vi "GlobalArm.vi"() -> ()   [LabVIEW 2020]
uses:
  <vilib>/robotics/Kinematics/Robot/NI_Robotics_Serial Robot Arm.lvclass
panel:
  out "SEN_Current_Wrist_Angle (deg)":dbl
  out "SEN_Current_Shoulder_Angle (deg)":dbl
  out "SEN_Current_Elbow_Angle (deg)":dbl
  out "OUT_Arm_Goal_Position (in)":dbl[](array[numeric])=[1.35, 0.0, 0.0]
  out "CON_Arm_Base_Position (in)":dbl[](array[numeric])=[1.35, 0.0, 0.0]
  out "CON_Gripper_Cone_Center_Of_Gravity (in)":dbl[](array[numeric])=[1.35, 0.0, 0.0]
  out "CON_Gripper_None_Center_Of_Gravity (in)":dbl[](array[numeric])=[1.35, 0.0, 0.0]
  out "CON_Forearm_Center_Of_Gravity (in)":dbl[](array[numeric])=[1.35, 0.0, 0.0]
  out "CON_Bicep_Center_Of_Gravity (in)":dbl[](array[numeric])=[1.35, 0.0, 0.0]
  out "CON_Gripper_Cone_Mass (lb)":dbl=1.0
  out "CON_Forearm_Mass (lb)":dbl=1.0
  out "CON_Bicep_Mass (lb)":dbl=1.0
  out "CON_Gripper_None_Mass (lb)":dbl=1.0
  out "CON_Forearm_Length (in)":dbl=1.0
  out "CON_Bicep_Length (in)":dbl=1.0
  out "CON_Gripper_Length (in)":dbl=1.0
  out "Serial_Arm_Cube":refnum<class "NI_Robotics_Serial Robot Arm.lvclass">
  out "Serial_Arm_Cone":refnum<class "NI_Robotics_Serial Robot Arm.lvclass">
  out "Serial_Arm_None":refnum<class "NI_Robotics_Serial Robot Arm.lvclass">
  out "SEN_Absolute_Wrist_Angle (deg)":dbl
  in  "OUT_Elbow_Mode":enum16{"Safety", "Travelling", "Positioning"}(ring)
  in  "OUT_Shoulder_Mode":enum16{"Safety", "Travelling", "Positioning"}(ring)
  in  "OUT_Wrist_Mode":enum16{"Safety", "Travelling", "Positioning"}(ring)
  out "SEN_Absolute_Shoulder_Angle (deg)":dbl
  out "SEN_Absolute_Elbow_Angle (deg)":dbl
  out "CON_Elbow_Gear_Ratio":dbl=1.0
  out "CON_Shoulder_Gear_Ratio":dbl=1.0
  out "CON_Wrist_Gear_Ratio":dbl=1.0
  out "OUT_Elbow_Goal (deg)":dbl
  out "OUT_Shoulder_Goal (deg)":dbl
  out "OUT_Wrist_Goal (deg)":dbl
  out "REF_Elbow":string
  out "REF_Shoulder":string
  out "REF_Wrist":string
  # "DEVICE REFERENCE NAMES"
  # "CONSTANTS"
  # "DRIVER STATION DATA"
  # "SENSORS"
  # "OUTPUTS"
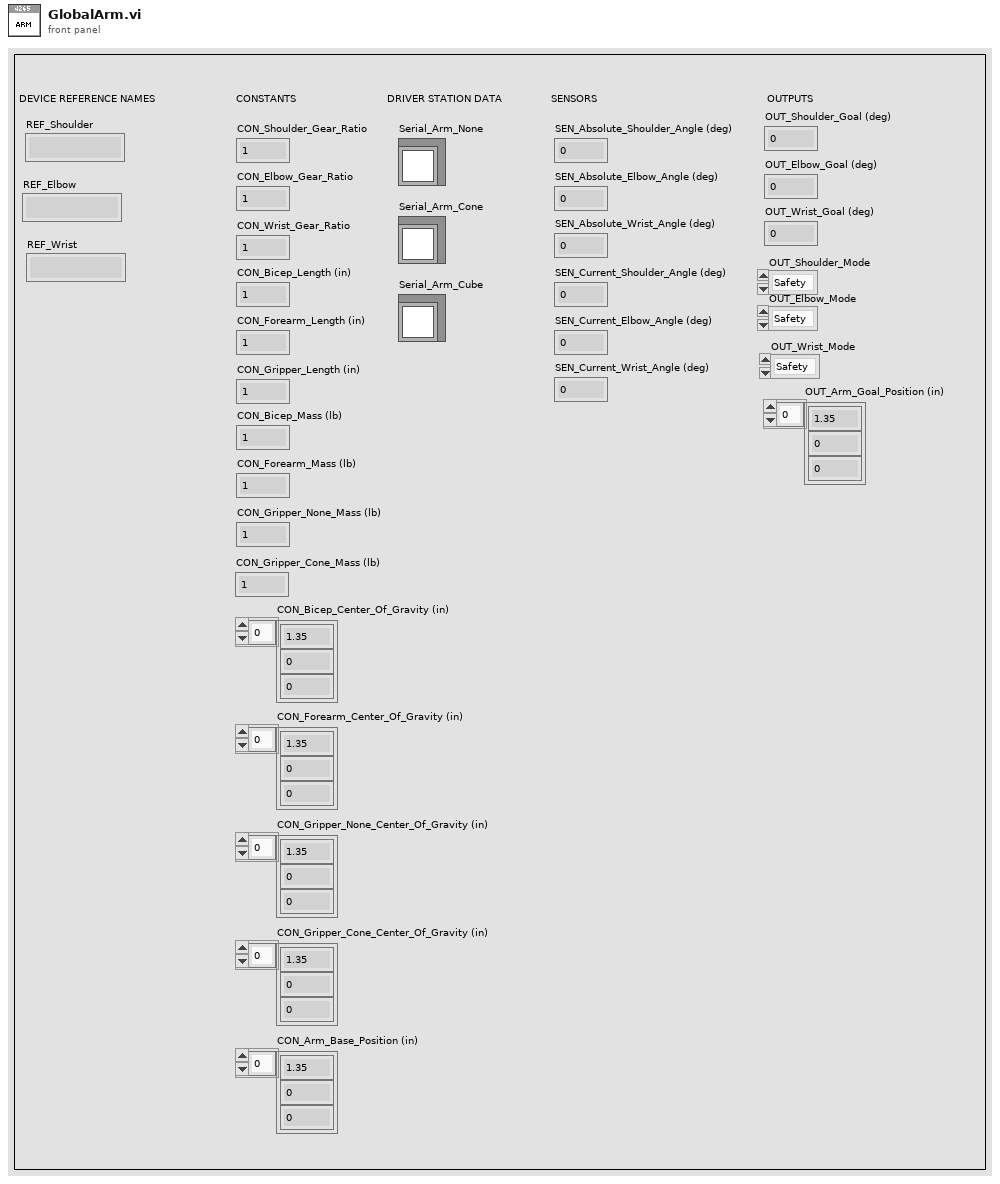
[diagram p1: front panel]
diagram:
